vi "CRYSet Graph Scale.vi"(6 "sOption":string, 8 "Flattened Property":string, 9 "Flattened Scale Property":string, 10 "pGraph In":refnum<vi>, 11 "pGraph VI In":refnum<vi>) -> (0 "Plot Settings":T1(array[cluster]), 3 "pGraph Out":refnum<vi>)   [LabVIEW 2013]
uses:
  Control/CRYGraph Scale.ctl
panel:
  in  "Graph Scale Property":T2={"X Scale.Maximum"=0.0, "X Scale.Minimum"=0.0, "Y0 Scale.Maximum"=0.0, "Y0 Scale.Minimum"=0.0, "Y1 Scale.Maximum"=0.0, "Y1 Scale.Minimum"=0.0, "X Scale.MapMode"=2, "Y1 Scale.MapMode"=2, "Y0 Scale.MapMode"=2, "ScaleFitX"=FALSE, "ScaleFitY"=FALSE, "ScaleFitY 2"=FALSE}
  in  "Plot Settings":T1(array[cluster])
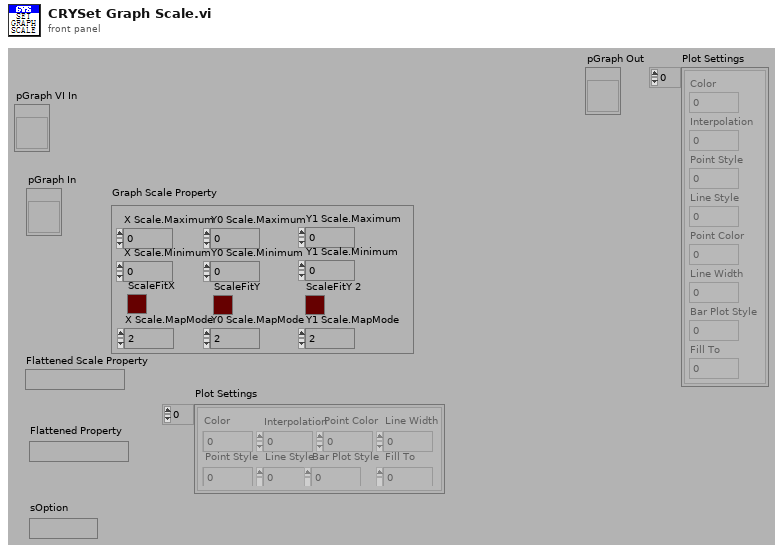
[diagram p1: front panel]
types:
  T1 = cluster{"Color":u32, "Interpolation":u8, "Point Style":u8, "Line Style":u8, "Point Color":u32, "Line Width":u8, "Bar Plot Style":u8, "Fill To":i16}[]
  T2 = typedef "CRYGraph Scale.ctl" = cluster{"X Scale.Maximum":dbl, "X Scale.Minimum":dbl, "Y0 Scale.Maximum":dbl, "Y0 Scale.Minimum":dbl, "Y1 Scale.Maximum":dbl, "Y1 Scale.Minimum":dbl, "X Scale.MapMode":u8, "Y1 Scale.MapMode":u8, "Y0 Scale.MapMode":u8, "ScaleFitX":bool, "ScaleFitY":bool, "ScaleFitY 2":bool}
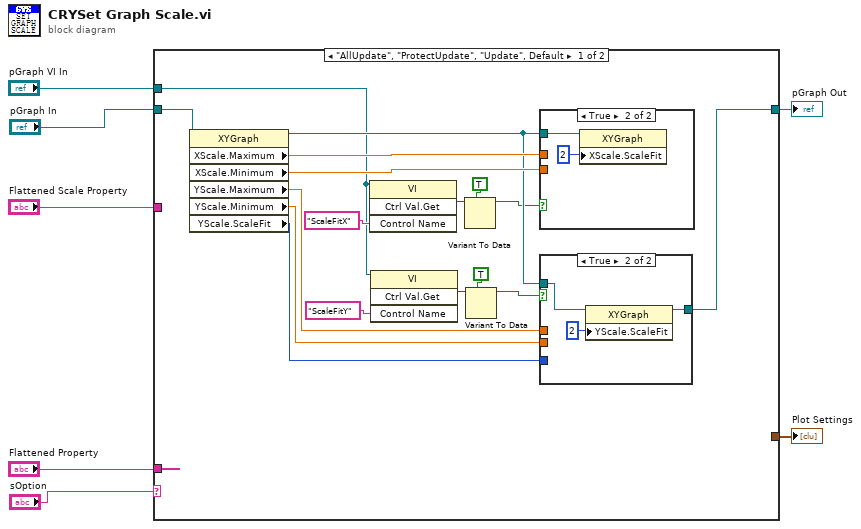
[diagram p0: block diagram]
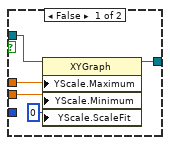
[diagram p2: hidden frame]
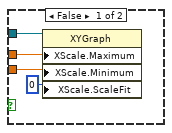
[diagram p3: hidden frame]
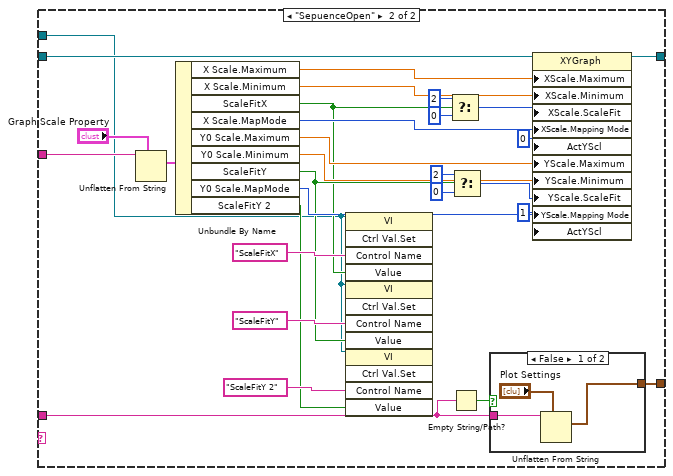
[diagram p4: hidden frame]
diagram:
  n1 = case shown="\"AllUpdate\", \"ProtectUpdate\", \"Update\", Default" "sOption" {
    tunnel: "pGraph In" -> [w24 w67]
    tunnel: [w18 w66] -> w2
    tunnel: "Flattened Scale Property" -> [_ w57]
    tunnel: [_ w53] -> w1
    tunnel: "Flattened Property" -> [_ w52]
    tunnel: "pGraph VI In" -> [w8 w39]
    frame "AllUpdate", "ProtectUpdate", "Update", Default {
      n2 = property class="XYGraph"(reference=w24) -> (reference out=w17:refnum<vi>, "XScale.Maximum"=w23:dbl, "XScale.Minimum"=w22:dbl, "YScale.Maximum"=w21:dbl, "YScale.Minimum"=w20:dbl, "YScale.ScaleFit"=w19:u8)  [unwired: 1 in, 1 out]
      n3 = invoke class="VI" method="Ctrl Val.Get"(reference=w8, "Control Name"="ScaleFitX") -> ("Get Control Value Variant"=w15:variant)  [unwired: 2 in, 3 out]
      n4 = invoke class="VI" method="Ctrl Val.Get"(reference=w8, "Control Name"="ScaleFitY") -> ("Get Control Value Variant"=w11:variant)  [unwired: 2 in, 3 out]
      n5 = Variant To Data(type=TRUE, Variant=w15) -> (data=w13:bool)  [unwired: 1 in, 1 out]
      n6 = Variant To Data(type=TRUE, Variant=w11) -> (data=w9:bool)  [unwired: 1 in, 1 out]
      n7 = case shown="True" w13 {
        tunnel: w23 -> [w36 _]
        tunnel: w22 -> [w35 _]
        tunnel: w17 -> [w34 w38]
        frame False {
          n8 = property class="XYGraph"(reference=w34, "XScale.Maximum"=w36, "XScale.Minimum"=w35, "XScale.ScaleFit"=u8 0 ("X Scale.Scale Fit")) -> ()  [unwired: 1 in, 2 out]
        }
        frame True {
          n9 = property class="XYGraph"(reference=w38, "XScale.ScaleFit"=u8 2 ("X Scale.Scale Fit")) -> ()  [unwired: 1 in, 2 out]
        }
      }
      n10 = case shown="True" w9 {
        tunnel: w17 -> [w29 w32]
        tunnel: [w28 w31] -> w18
        tunnel: w21 -> [w27 _]
        tunnel: w20 -> [w26 _]
        tunnel: w19 -> [_ _]
        frame False {
          n11 = property class="XYGraph"(reference=w29, "YScale.Maximum"=w27, "YScale.Minimum"=w26, "YScale.ScaleFit"=u8 0 ("Y Scale.Scale Fit")) -> (reference out=w28:refnum<vi>)  [unwired: 1 in, 1 out]
        }
        frame True {
          n12 = property class="XYGraph"(reference=w32, "YScale.ScaleFit"=u8 2 ("Y Scale.Scale Fit")) -> (reference out=w31:refnum<vi>)  [unwired: 1 in, 1 out]
        }
      }
    }
    frame "SepuenceOpen" {
      n13 = Unflatten From String(type="Graph Scale Property", binary string=w57) -> (value=w56:T2)  [unwired: 3 in, 2 out]
      n14 = Unbundle By Name(w56) -> ("X Scale.Maximum"=w63:dbl, "X Scale.Minimum"=w62:dbl, "ScaleFitX"=w40:bool, "X Scale.MapMode"=w59:u8, "Y0 Scale.Maximum"=w61:dbl, "Y0 Scale.Minimum"=w60:dbl, "ScaleFitY"=w41:bool, "Y0 Scale.MapMode"=w58:u8, "ScaleFitY 2"=w42:bool)
      n15 = invoke class="VI" method="Ctrl Val.Set"(reference=w39, "Control Name"="ScaleFitX", "Value"=w40) -> ()  [unwired: 2 in, 5 out]
      n16 = invoke class="VI" method="Ctrl Val.Set"(reference=w39, "Control Name"="ScaleFitY", "Value"=w41) -> ()  [unwired: 2 in, 5 out]
      n17 = invoke class="VI" method="Ctrl Val.Set"(reference=w39, "Control Name"="ScaleFitY 2", "Value"=w42) -> ()  [unwired: 2 in, 5 out]
      n18 = Select(t=u8 2, s=w40, f=u8 0 ("X Scale.Scale Fit")) -> (s? t:f=w50:u8)
      n19 = Empty String/Path?(string/path=w52) -> (empty?=w54:bool)
      n20 = Select(t=u8 2, s=w41, f=u8 0 ("X Scale.Scale Fit")) -> (s? t:f=w47:u8)
      n21 = case shown="False" w54 {
        tunnel: w52 -> [w70 _]
        tunnel: [w68 _] -> w53
        frame False {
          n22 = Unflatten From String(type="Plot Settings", binary string=w70) -> (value=w68:T1)  [unwired: 3 in, 2 out]
        }
        frame True {
        }
      }
      n23 = property class="XYGraph"(reference=w67, "XScale.Maximum"=w63, "XScale.Minimum"=w62, "XScale.ScaleFit"=w50, "XScale.Mapping Mode"=w59, "ActYScl"=0 ("Active Y Scale"), "YScale.Maximum"=w61, "YScale.Minimum"=w60, "YScale.ScaleFit"=w47, "YScale.Mapping Mode"=w58, "ActYScl"=1 ("Active Y Scale")) -> (reference out=w66:refnum<vi>)  [unwired: 1 in, 1 out]
    }
  }
  "pGraph Out" <- w2
  "Plot Settings" <- w1
